vi "DeltaFbyF.vi"(9 "Data in":T1) -> (1 "Data out":T1)   [LabVIEW 2013]
uses:
  xcontrol/Interface VIs/Interface typedefs/Interface-Data array.ctl
  xcontrol/Interface VIs/Interface typedefs/Interface-Data format definition.ctl
  xcontrol/Typedefs/Xctl-XY data type definition.ctl
  xcontrol/Typedefs/Xctrl-ROI type enum.ctl
  <vilib>/Analysis/baseanly.llb/Mean (DBL).vi
  Global variables/gl_Functional Imaging-Global variables.vi
  <vilib>/Analysis/NI_AALBase.lvlib
  xcontrol/XGrapher.xctl
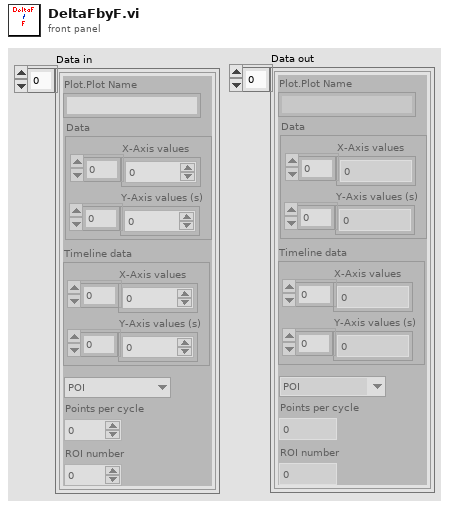
[diagram p1: front panel]
types:
  T1 = typedef "Interface-Data array.ctl" = T2[]
  T2 = typedef "Interface-Data format definition.ctl" = cluster{"Plot.Plot Name":string, "Data":T3, "Timeline data":T3, "Type":T4, "Points per cycle":u16, "ROI number":u16}
  T3 = typedef "XGrapher.xctl/Xctl-XY data type definition.ctl" = cluster{"X-Axis values":sgl[], "Y-Axis values (s)":i32[]}
  T4 = typedef "Xctrl-ROI type enum.ctl" = enum16{"POI", "Mini-scan", "Group"}
  T5 = typedef "Functional Imging UI Refs.ctl" = cluster{"Menu ref":refnum<k9>, "Image control":refnum<vi>, "VI ref":refnum<vi>, "XGrapher":refnum<vi>, "Smoothing":refnum<vi>, "POI Averaging":refnum<vi>, "Normalize":refnum<vi>, "POI data points in each trial":refnum<vi>, "Channel":refnum<vi>, "Experiment data folder path":refnum<vi>, "[ROI vis]":refnum<vi>, "[Groups] visbl":T6, "Group Name":refnum<vi>, "POI index":refnum<vi>, "Trial No.":refnum<vi>, "Intensity Zoom":refnum<vi>, "Trial Cursor Enabled":refnum<vi>, "Number of Trials (ind 1)":refnum<vi>, "Number of Trials (ind 2)":refnum<vi>, "MiniScans Available":refnum<vi>, "POI Available":refnum<vi>, "Defer graph updates":refnum<vi>, "Waveform selector":refnum<vi>, "#of selected POI":refnum<vi>, "#of selected MiniScans":refnum<vi>, "#of selected groups":refnum<vi>, "Max Z-Projection":refnum<vi>, "Z-Plane Selector":refnum<vi>, "Index of miniscan point to visualise":refnum<vi>, "ROI vis. mode":refnum<vi>, "Total # of points":refnum<vi>, "Index of group clicked on":refnum<vi>, "Pane 1":refnum<vi>, "Pane 2":refnum<vi>, "Pane 3":refnum<vi>, "Pane 4":refnum<vi>, "Pane 5":refnum<vi>, "Pane 6":refnum<vi>, "Deselect all ROI":refnum<vi>, "Deselect all groups":refnum<vi>}
  T6 = typedef "Groups array referecne.ctl" = refnum<vi>
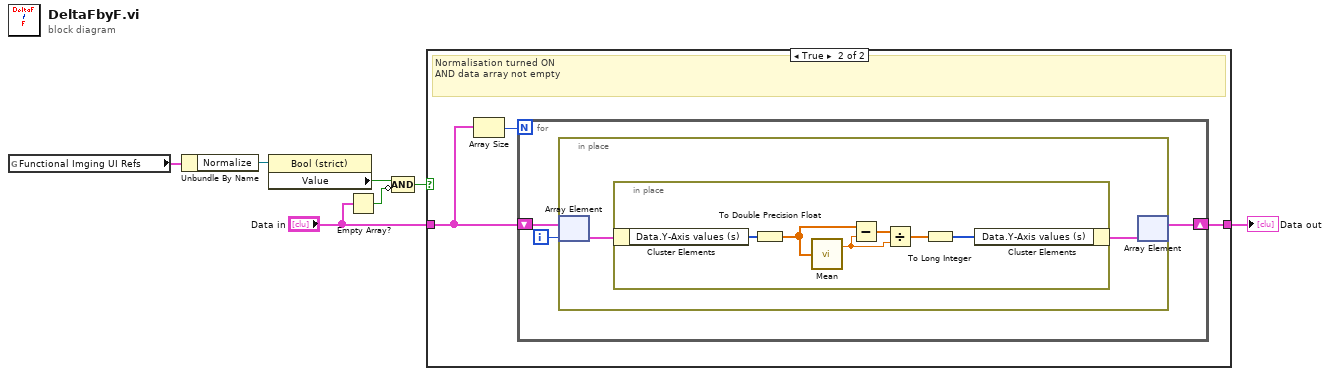
[diagram p0: block diagram]
diagram:
  n1 = global read "gl_Functional Imaging-Global variables.vi" "Functional Imging UI Refs"() -> (w1:T5)
  n2 = Unbundle By Name(w1) -> ("Normalize"=w7:refnum<vi>)
  n3 = property on="Property Node" class="Bool (strict)"(reference=w7) -> ("Value"=w5:bool)  [unwired: 1 in, 2 out]
  n4 = Empty Array?(array="Data in") -> (empty?=w6:bool)
  n5 = Compound Arithmetic op=AND(w5, invert w6) -> (w4:bool)
  n6 = case shown="True" w4 {
    tunnel: "Data in" -> [w8 w9]
    tunnel: [w8 w11] -> w2
    frame False {
      # "Normalisation turned OFF\nOR no data array is empty"
    }
    frame True {
      # "Normalisation turned ON\nAND data array not empty"
      n7 = Array Size(array=w9) -> (size(s)=w10:i32)
      n8 = for {
        N: w10 -> [_]
        shift-right: [w13] -> w11
        shift-left: w9 -> [w12]
        i -> [w14]
        n9 = in-place {
          n10 = in-place-array #1(w12, w14) -> (w16:T2)
          n11 = in-place {
            n12 = in-place-cluster #2(w16) -> ("Data.Y-Axis values (s)"=w20:i32[])
            n13 = To Double Precision Float(number=w20) -> (double precision float=w18:dbl[])
            n14 = call-poly <vilib>:"Mean.vi"("X"=w18) -> ("mean"=w21:dbl)  [unwired: 1 out]
            n15 = Subtract(x=w18, y=w21) -> (x-y=w22:dbl[])
            n16 = Divide(x=w22, y=w21) -> (x/y=w19:dbl[])
            n17 = To Long Integer(number=w19) -> (32bit integer=w17:i32[])
            n18 = in-place-cluster #2("Data.Y-Axis values (s)"=w17) -> (w15:T2)
          }
          n19 = in-place-array #1(w15) -> (w13:T1)  [unwired: 1 out]
        }
      }
    }
  }
  "Data out" <- w2
